vi "RAMP_close_single_scan.vi"(1 "queue ASI stage":refnum<queue>, 5 "queue CAMERA":refnum<queue>, 9 "queue piezo":refnum<queue>, 11 "error in":errorcluster, 12 "Z_position_file path":path, 14 "Illumination source":bool) -> (15 "error out":errorcluster)   [LabVIEW 2015]
uses:
  CONTROLS/Q_ASI_stage_element.ctl
  CONTROLS/Q_MCL_piezo_element.ctl
  CONTROLS/Q_camera_element.ctl
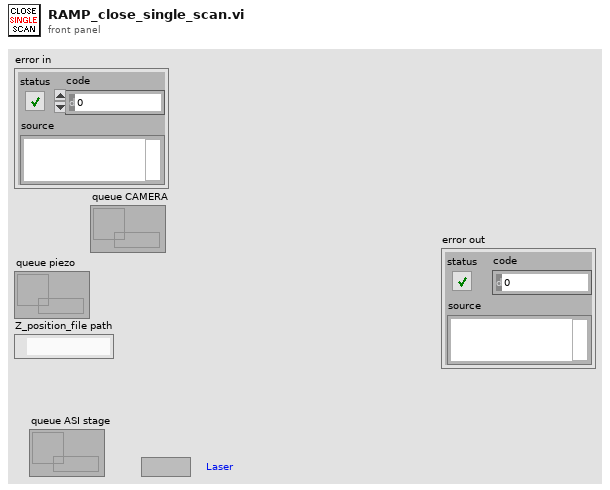
[diagram p1: front panel]
types:
  T1 = typedef "Q_camera_element.ctl" = cluster{"variant":variant, "Instruction":enum16{"CAMERA_idle", "CAMERA_initialize", "CAMERA_error", "CAMERA_security_stop", "CAMERA_not_acquiring", "CAMERA_acquiring", "CAMERA_start_acquiring", "CAMERA_stop_acquiring", "CAMERA_change_exposure", "CAMERA_define_ROI", "CAMERA_cooler", "CAMERA_acquire_movie", "CAMERA_init_scan", "CAMERA_check_new_scan_image", "CAMERA_close_scan", "CAMERA_init_merFISH", "CAMERA_start_acquiring_merFISH", "CAMERA_close_scan_merFISH", "CAMERA_close_merFISH", "CAMERA_init_TL", "CAMERA_start_acquiring_TL", "CAMERA_stop_acquiring_TL", "CAMERA_close_TL", "CAMERA_STOP"}}
  T2 = typedef "Q_MCL_piezo_element.ctl" = cluster{"variant":variant, "Instruction":enum16{"Piezo_idle", "Piezo_initialize", "Piezo_error", "Piezo_security_stop", "Piezo_read_z", "Piezo_move_z", "Piezo_keyboard_move", "Piezo_close_autofocus_calibration_ramp", "Piezo_change_init_state", "Piezo_init_autofocus", "Piezo_init_autofocus_merFISH_TL", "Piezo_autofocus", "Piezo_autofocus_merFISH_TL", "Piezo_stop_autofocus", "Piezo_stop_autofocus_merFISH_TL", "Piezo_autofocus_lost", "Piezo_resume_autofocus_merFISH_TL", "Piezo_check_z_position_merFISH_TL", "Piezo_init_ramp", "Piezo_move_z_ramp", "Piezo_close_ramp", "Piezo_close_merFISH", "Piezo_stop"}}
  T3 = typedef "Q_ASI_stage_element.ctl" = cluster{"variant":variant, "Instruction":enum16{"ASI_idle", "ASI_initialize", "ASI_error", "ASI_security_stop", "ASI_read_XYZ", "ASI_up", "ASI_down", "ASI_left", "ASI_right", "ASI_save_XY", "ASI_move_to_XY", "ASI_brightfield", "ASI_init_scan", "ASI_init_merFISH", "ASI_move_to_XY_merFISH", "ASI_move_to_Z_merFISH", "ASI_init_autofocus_search_merFISH", "ASI_close_autofocus_search_merFISH", "ASI_adjust_piezo_autofocus_merFISH", "ASI_set_piezo_autofocus_to_reference_position_merFISH_TL", "ASI_close_merFISH", "ASI_stop"}}
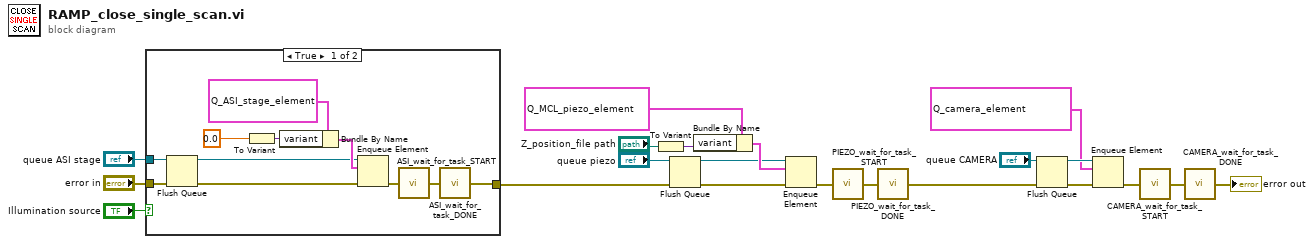
[diagram p0: block diagram]
diagram:
  n1 = case shown="True" "Illumination source" {
    tunnel: "error in" -> [w32 w33]
    tunnel: "queue ASI stage" -> [w31 _]
    tunnel: [w22 w33] -> w13
    frame True {
      n2 = Flush Queue(queue=w31, error in (no error)=w32) -> (queue out=w25:refnum<queue>, error out=w27:errorcluster)  [unwired: 1 out]
      n3 = To Variant(anything=0.0) -> (Variant=w29:variant)
      n4 = Bundle By Name(cluster=T3 {"variant"=variant, "Instruction"=enum."ASI_brightfield"} ("Q_ASI_stage"), "variant"=w29) -> (w26:T3)
      n5 = Enqueue Element(queue=w25, element=w26, error in (no error)=w27) -> (error out=w24:errorcluster)  [unwired: 1 in, 2 out]
      n6 = call "ASI_wait_for_task_START.vi"("error in"=w24) -> ("error out"=w23:errorcluster)
      n7 = call "ASI_wait_for_task_DONE.vi"("error in"=w23) -> ("error out"=w22:errorcluster)
    }
    frame False {
    }
  }
  n8 = To Variant(anything="Z_position_file path") -> (Variant=w12:variant)
  n9 = Flush Queue(queue="queue piezo", error in (no error)=w13) -> (queue out=w14:refnum<queue>, error out=w17:errorcluster)  [unwired: 1 out]
  n10 = Bundle By Name(cluster=T2 {"variant"=variant, "Instruction"=enum."Piezo_close_ramp"} ("Q_MCL_Piezo"), "variant"=w12) -> (w15:T2)
  n11 = Enqueue Element(queue=w14, element=w15, error in (no error)=w17) -> (error out=w10:errorcluster)  [unwired: 1 in, 2 out]
  n12 = call "PIEZO_wait_for_task_START.vi"("error in"=w10) -> ("error out"=w9:errorcluster)
  n13 = call "PIEZO_wait_for_task_DONE.vi"("error in"=w9) -> ("error out"=w4:errorcluster)
  n14 = Flush Queue(queue="queue CAMERA", error in (no error)=w4) -> (queue out=w6:refnum<queue>, error out=w5:errorcluster)  [unwired: 1 out]
  n15 = Enqueue Element(queue=w6, element=T1 {"variant"=variant, "Instruction"=enum."CAMERA_close_scan"} ("Q_ANDOR_element"), error in (no error)=w5) -> (error out=w7:errorcluster)  [unwired: 1 in, 2 out]
  n16 = call "CAMERA_wait_for_task_START.vi"("error in"=w7) -> ("error out"=w8:errorcluster)
  n17 = call "CAMERA_wait_for_task_DONE.vi"("error in"=w8) -> ("error out"=→"error out":errorcluster)
